vi "FPGA_controller.vi"() -> ()   [LabVIEW 2017]
uses:
  <vilib>/rvi/Emulation/niFpgaGetClockAttributes.vi
  <vilib>/rvi/Emulation/niFpgaSctlEmulationGetInTimedLoop.vi
  <vilib>/rvi/Emulation/niFpgaEmulationReportErrorSimple.vi
  <vilib>/rvi/eio/common/nirviEmuTemplateMethod_errors.vi
  <vilib>/rvi/Emulation/niFpgaCriticalErrorInLSC.vi
  <vilib>/eio/EIONode/EIONode.xnode
panel:
  out "VALID":bool
  in  "m_first u2":fxp<+/-,64,32>=-0.8999999999068677 format="%#_42g"
  in  "m_first u1":fxp<+/-,64,32>=-0.8999999999068677 format="%#_42g"
  in  "Scale u2":fxp<+/-,64,42>=5.0 format="%#_35g"
  in  "Offset u2":fxp<+/-,64,41>=2.0 format="%#_36g"
  in  "Scale u1":fxp<+/-,64,42>=5.0 format="%#_35g"
  in  "Offset u1":fxp<+/-,64,41>=2.0 format="%#_36g"
  in  "eta u":fxp<+,16,1>=0.29998779296875 format="%#_42g"
  in  "Scale x2":fxp<+/-,32,16>=10.0 format="%#_21g"
  in  "m_first x2":fxp<+/-,49,33> format="%#_26g"
  in  "Offset x2":fxp<+/-,48,32> format="%#_26g"
  in  "Offset x3":fxp<+/-,48,32>=5.0 format="%#_26g"
  in  "m_first x3":fxp<+/-,32,16>=-3.399993896484375 format="%#_21g"
  in  "Scale x3":fxp<+/-,32,16>=10.0 format="%#_21g"
  in  "1/eta x":fxp<+,3,3>=5.0 format="%#_21g"
  in  "m_first x1":fxp<+/-,49,33> format="%#_26g"
  in  "Offset x1":fxp<+/-,48,32> format="%#_26g"
  in  "Scale x1":fxp<+/-,32,16>=10.0 format="%#_21g"
  in  "stop":bool
  # "INPUTS CONVERSION"
  # "STATES CONVERSION"
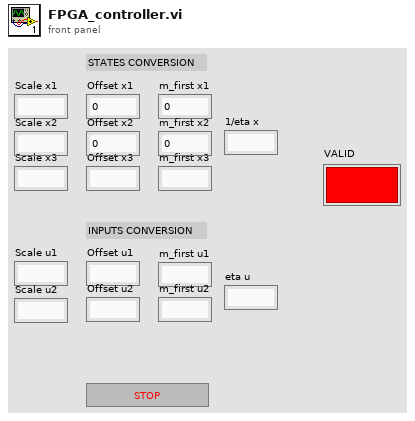
[diagram p1: front panel]
types:
  T1 = cluster{"Boolean array[0]":bool, "Boolean array[1]":bool, "Boolean array[2]":bool, "Boolean array[3]":bool, "Boolean array[4]":bool, "Boolean array[5]":bool, "Boolean array[6]":bool, "Boolean array[7]":bool, "Boolean array[8]":bool, "Boolean array[9]":bool, "Boolean array[10]":bool, "Boolean array[11]":bool, "Boolean array[12]":bool, "Boolean array[13]":bool, "Boolean array[14]":bool, "Boolean array[15]":bool, "Boolean array[16]":bool, "Boolean array[17]":bool}
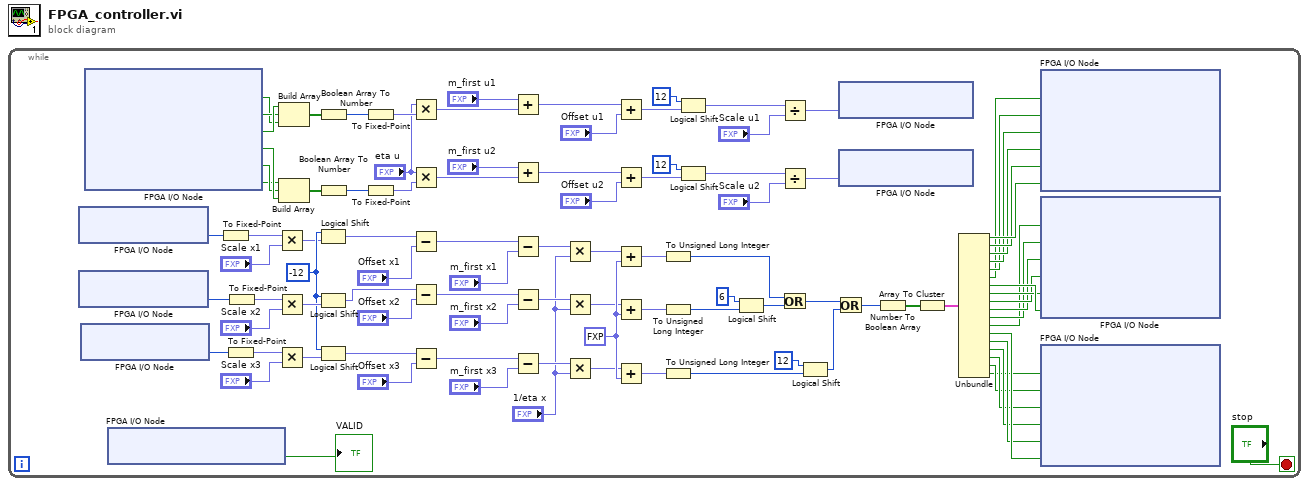
[diagram p0: block diagram]
diagram:
  n1 = while {
    stop <- "stop" stop-if-true
    w38 = fxp<+,2,1> 0.5 ("y")
    w31 = i16 -12 ("y")
    n2 = xnode "FPGA I/O Node"() -> ("ConnectorA/AI0"=w6:u16)  [unwired: 1 in, 1 out]
    n3 = xnode "FPGA I/O Node"() -> ("ConnectorA/AI1"=w4:u16)  [unwired: 1 in, 1 out]
    n4 = xnode "FPGA I/O Node"() -> ("ConnectorB/AI0"=w2:u16)  [unwired: 1 in, 1 out]
    n5 = xnode "FPGA I/O Node"() -> ("Component-Level IP\\po0"=w95:bool, "Component-Level IP\\po1"=w96:bool, "Component-Level IP\\po2"=w97:bool, "Component-Level IP\\po3"=w72:bool, "Component-Level IP\\po4"=w71:bool, "Component-Level IP\\po5"=w70:bool)  [unwired: 6 in, 6 out]
    n6 = xnode "FPGA I/O Node"() -> ("Component-Level IP\\po6"=→"VALID":bool)  [unwired: 1 in, 1 out]
    n7 = To Fixed-Point(number=w6) -> (fixed-point=w5:fxp<+,16,16>)  [unwired: 1 in]
    n8 = To Fixed-Point(number=w2) -> (fixed-point=w1:fxp<+,16,16>)  [unwired: 1 in]
    n9 = To Fixed-Point(number=w4) -> (fixed-point=w3:fxp<+,16,16>)  [unwired: 1 in]
    n10 = Multiply(x=w5, y="Scale x1") -> (x*y=w22:fxp<+/-,48,32>)
    n11 = Multiply(x=w3, y="Scale x2") -> (x*y=w40:fxp<+/-,48,32>)
    n12 = Multiply(x=w1, y="Scale x3") -> (x*y=w28:fxp<+/-,48,32>)
    n13 = Build Array(w97, w96, w95) -> (w93:bool[])
    n14 = Build Array(w70, w71, w72) -> (w81:bool[])
    n15 = Logical Shift(y=w31, x=w22) -> (x << y=w18:fxp<+/-,48,32>)
    n16 = Logical Shift(y=w31, x=w40) -> (x << y=w12:fxp<+/-,48,32>)
    n17 = Logical Shift(y=w31, x=w28) -> (x << y=w27:fxp<+/-,48,32>)
    n18 = Boolean Array To Number(Boolean array=w93) -> (number=w89:u8)
    n19 = Boolean Array To Number(Boolean array=w81) -> (number=w78:u8)
    n20 = To Fixed-Point(number=w89) -> (fixed-point=w88:fxp<+,8,8>)  [unwired: 1 in]
    n21 = To Fixed-Point(number=w78) -> (fixed-point=w77:fxp<+,8,8>)  [unwired: 1 in]
    n22 = Multiply(x="eta u", y=w88) -> (x*y=w94:fxp<+,24,9>)
    n23 = Multiply(x="eta u", y=w77) -> (x*y=w82:fxp<+,24,9>)
    n24 = Subtract(x=w18, y="Offset x1") -> (x-y=w19:fxp<+/-,49,33>)
    n25 = Subtract(x=w12, y="Offset x2") -> (x-y=w14:fxp<+/-,49,33>)
    n26 = Subtract(x=w27, y="Offset x3") -> (x-y=w29:fxp<+/-,49,33>)
    n27 = Add(x="m_first u1", y=w94) -> (x+y=w92:fxp<+/-,64,33>)
    n28 = Add(x="m_first u2", y=w82) -> (x+y=w80:fxp<+/-,64,33>)
    n29 = Subtract(x=w19, y="m_first x1") -> (x-y=w21:fxp<+/-,50,34>)
    n30 = Subtract(x=w14, y="m_first x2") -> (x-y=w11:fxp<+/-,50,34>)
    n31 = Subtract(x=w29, y="m_first x3") -> (x-y=w35:fxp<+/-,50,34>)
    n32 = Multiply(x=w21, y="1/eta x") -> (x*y=w16:fxp<+/-,53,37>)
    n33 = Multiply(x=w11, y="1/eta x") -> (x*y=w9:fxp<+/-,53,37>)
    n34 = Multiply(x=w35, y="1/eta x") -> (x*y=w34:fxp<+/-,52,36>)
    n35 = Add(x=w92, y="Offset u1") -> (x+y=w87:fxp<+/-,64,42>)
    n36 = Add(x=w80, y="Offset u2") -> (x+y=w76:fxp<+/-,64,42>)
    n37 = Add(x=w16, y=w38) -> (x+y=w49:fxp<+/-,53,37>)
    n38 = Add(x=w9, y=w38) -> (x+y=w37:fxp<+/-,53,37>)
    n39 = Add(x=w34, y=w38) -> (x+y=w36:fxp<+/-,52,36>)
    n40 = To Unsigned Long Integer(number=w49) -> (unsigned 32bit integer=w45:u32)
    n41 = To Unsigned Long Integer(number=w37) -> (unsigned 32bit integer=w47:u32)
    n42 = To Unsigned Long Integer(number=w36) -> (unsigned 32bit integer=w43:u32)
    n43 = Logical Shift(y=i16 12, x=w87) -> (x << y=w85:fxp<+/-,64,42>)
    n44 = Logical Shift(y=i16 12, x=w76) -> (x << y=w74:fxp<+/-,64,42>)
    n45 = Logical Shift(y=6, x=w47) -> (x << y=w46:u32)
    n46 = Divide(x=w85, y="Scale u1") -> (x/y=w83:fxp<+/-,64,65>)
    n47 = Divide(x=w74, y="Scale u2") -> (x/y=w73:fxp<+/-,64,65>)
    n48 = Or(x=w45, y=w46) -> (x .or. y?=w41:u32)
    n49 = Logical Shift(y=12, x=w43) -> (x << y=w42:u32)
    n50 = Or(x=w41, y=w42) -> (x .or. y?=w26:u32)
    n51 = xnode "FPGA I/O Node"("ConnectorB/AO0"=w83) -> ()  [unwired: 1 in, 1 out]
    n52 = xnode "FPGA I/O Node"("ConnectorB/AO1"=w73) -> ()  [unwired: 1 in, 1 out]
    n53 = Number To Boolean Array(number=w26) -> (Boolean array=w50:bool[])
    n54 = Array To Cluster(array=w50) -> (cluster=w69:T1)
    n55 = Unbundle(w69) -> ("Boolean array[0]"=w68:bool, "Boolean array[1]"=w67:bool, "Boolean array[2]"=w66:bool, "Boolean array[3]"=w65:bool, "Boolean array[4]"=w64:bool, "Boolean array[5]"=w63:bool, "Boolean array[6]"=w62:bool, "Boolean array[7]"=w61:bool, "Boolean array[8]"=w60:bool, "Boolean array[9]"=w59:bool, "Boolean array[10]"=w58:bool, "Boolean array[11]"=w57:bool, "Boolean array[12]"=w56:bool, "Boolean array[13]"=w55:bool, "Boolean array[14]"=w54:bool, "Boolean array[15]"=w53:bool, "Boolean array[16]"=w52:bool, "Boolean array[17]"=w51:bool)
    n56 = xnode "FPGA I/O Node"("Component-Level IP\\pi00"=w63, "Component-Level IP\\pi01"=w64, "Component-Level IP\\pi02"=w65, "Component-Level IP\\pi03"=w66, "Component-Level IP\\pi04"=w67, "Component-Level IP\\pi05"=w68) -> ()  [unwired: 6 in, 6 out]
    n57 = xnode "FPGA I/O Node"("Component-Level IP\\pi06"=w57, "Component-Level IP\\pi07"=w58, "Component-Level IP\\pi08"=w59, "Component-Level IP\\pi09"=w60, "Component-Level IP\\pi10"=w61, "Component-Level IP\\pi11"=w62) -> ()  [unwired: 6 in, 6 out]
    n58 = xnode "FPGA I/O Node"("Component-Level IP\\pi12"=w51, "Component-Level IP\\pi13"=w52, "Component-Level IP\\pi14"=w53, "Component-Level IP\\pi15"=w54, "Component-Level IP\\pi16"=w55, "Component-Level IP\\pi17"=w56) -> ()  [unwired: 6 in, 6 out]
  }
